vi "Global 3.vi"() -> ()   [LabVIEW 2023]
panel:
  in  "stop":bool
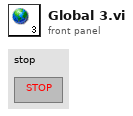
[diagram p1: front panel]
diagram:
